vi "LABVIEW_Simulare_Adaptiv_Iluminare_Autovehicul.vi"() -> ()   [LabVIEW 2020]
panel:
  out "Volan - Faruri UNGHI":dynamicdata(graph)
  out "Viteza":dbl(graph)
  out "Grafic stari faza lunga/scurta":i32(graph)
  out "Grafic stari lumini ceata":i32(graph)
  in  "lceata":bool
  in  "?":bool
  in  "?":bool
  in  "Checkbox pt masina fata/localitate":bool
  in  "UMIDITATE":dbl(slide) scale=0.0..100.0
  in  "VITEZA":dbl(slide) scale=0.0..250.0
  out "Pozitionare Faruri":dbl(knob) scale=60.0..120.0
  in  "flunga":bool
  in  "fscurta":bool
  in  "?":bool
  in  "VOLAN":dbl(knob) scale=45.0..135.0
  out "ceata":bool
  out "adaptiv":bool
  out "fscurta":bool
  out "flunga":bool
  out "Vitezometru":dbl(knob) scale=0.0..250.0
  # "stare 0 -  Manual     oprit\nstare 1 -  Manual     f scurta\nstare 2 -  Manual     f scurta+lunga\nstare 3 -  Automat  f scurta\nstare 4 -  Automat  f scurta+lunga"
  # "stare 0 -  Oprit   \nstare 1 -  Manual\nstare 2 -  Automat"
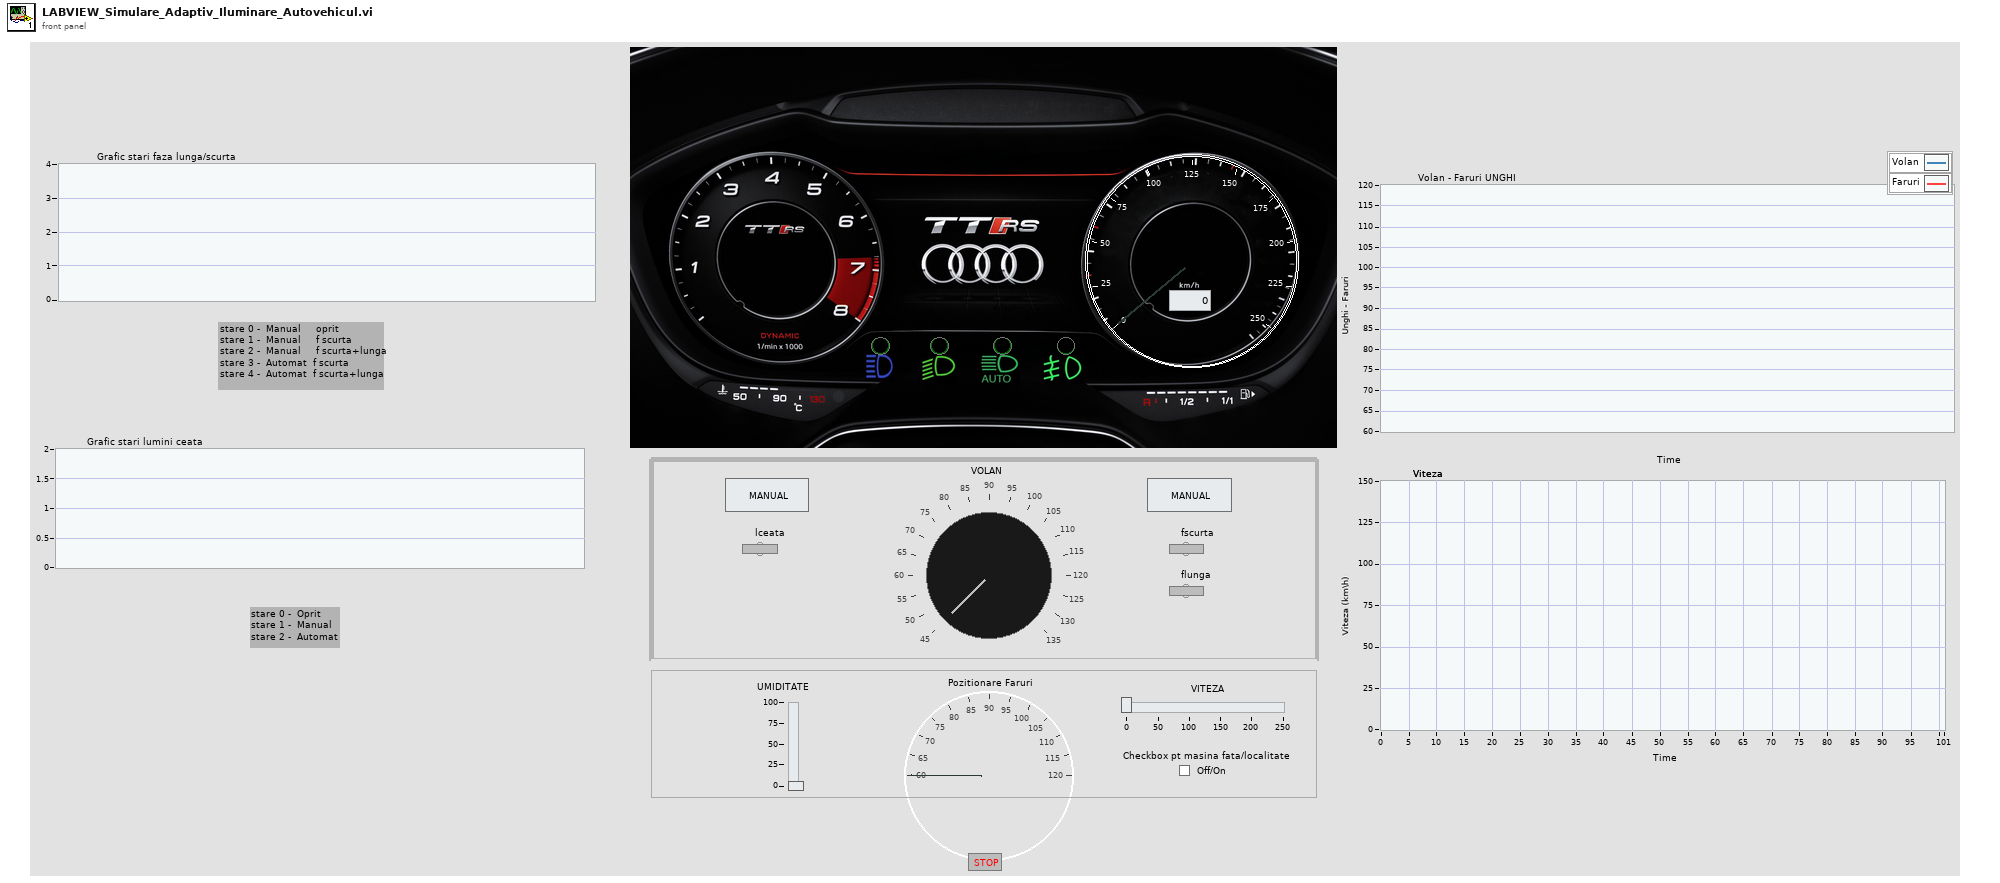
[diagram p1: front panel]
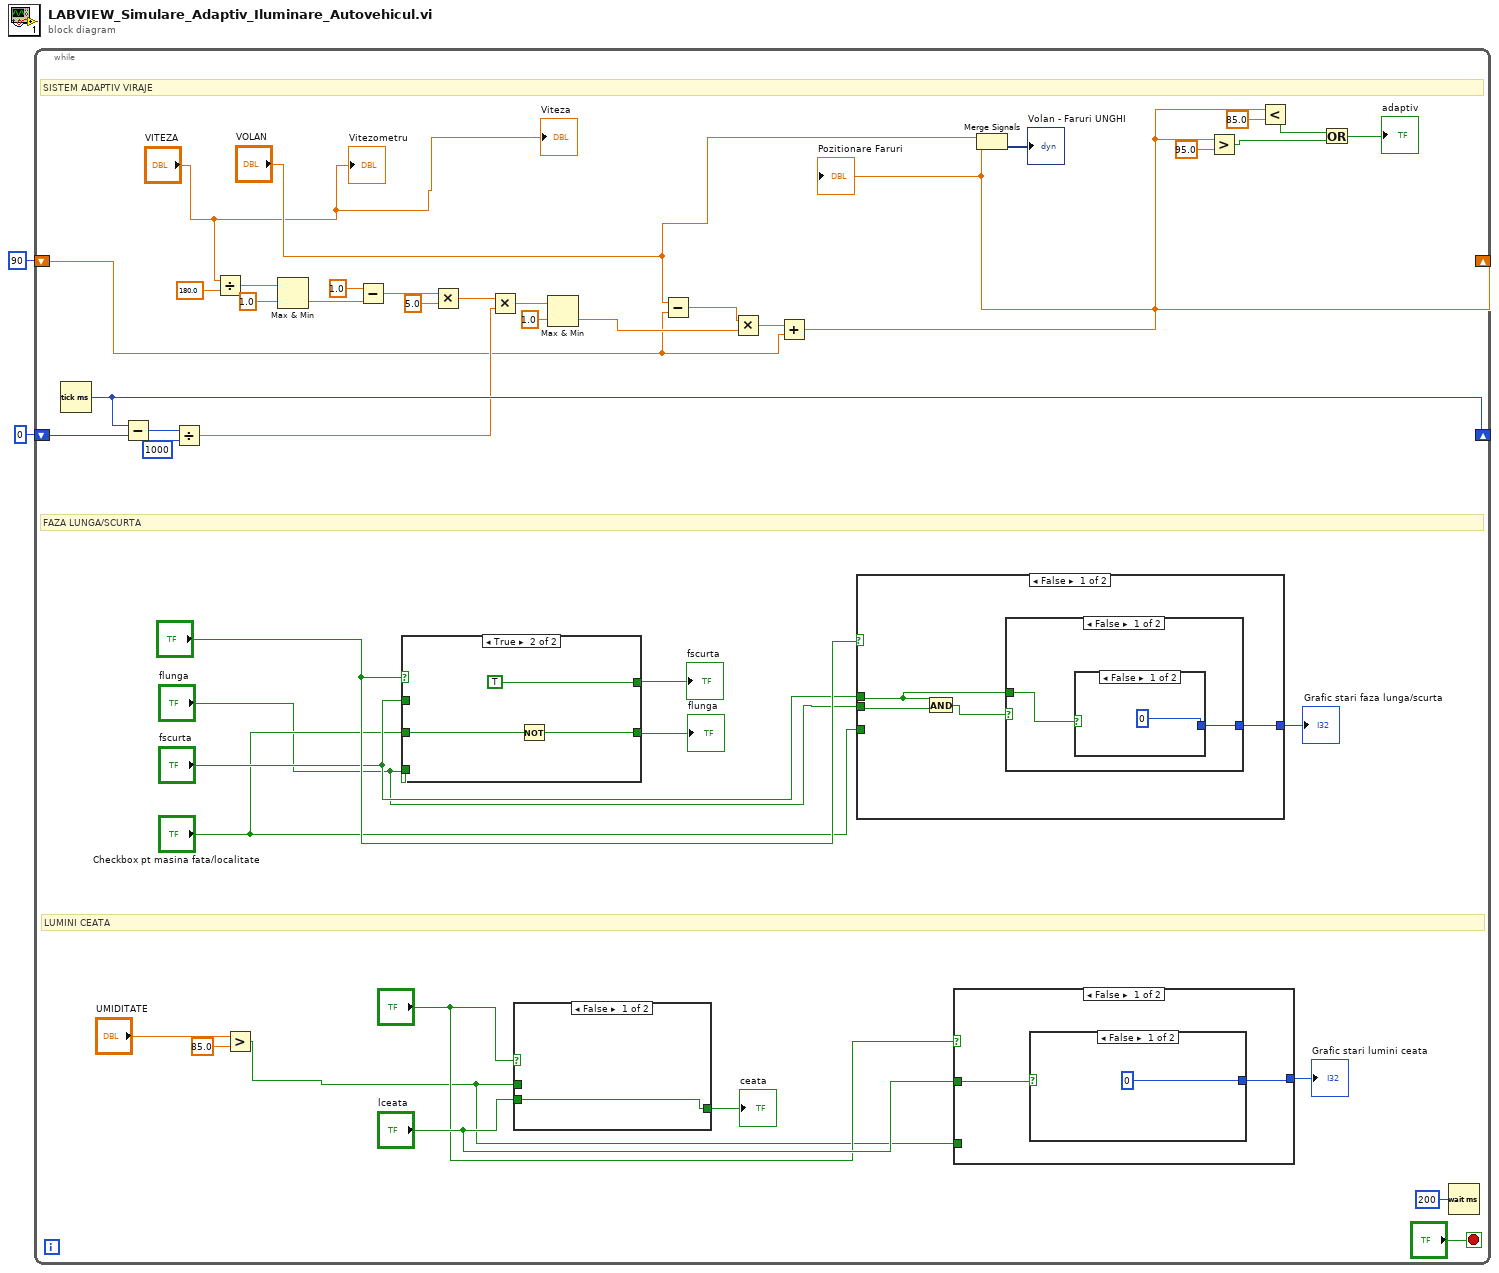
[diagram p0: block diagram]
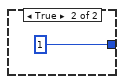
[diagram p2: hidden frame]
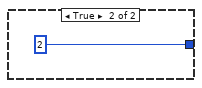
[diagram p3: hidden frame]
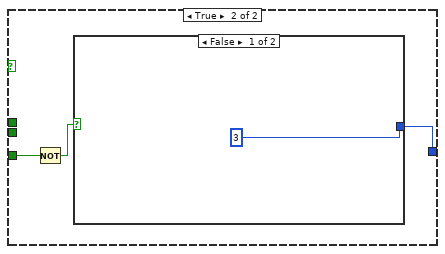
[diagram p4: hidden frame]
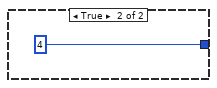
[diagram p5: hidden frame]
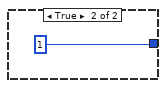
[diagram p7: hidden frame]
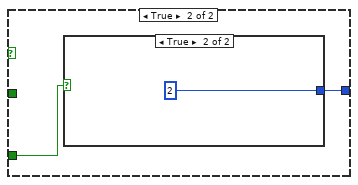
[diagram p8: hidden frame]
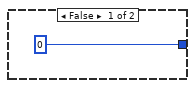
[diagram p9: hidden frame]
diagram:
  n1 = while {
    shift-right: [w6] -> _
    shift-left: 90 -> [w26]
    shift-right: [w41] -> _
    shift-left: 0 -> [w44]
    stop <- "?" stop-if-true
    # "LUMINI CEATA"
    # "FAZA LUNGA/SCURTA"
    # "SISTEM ADAPTIV VIRAJE"
    n2 = Tick Count (ms)() -> (millisecond timer value=w41:u32)
    n3 = Subtract(x=w41, y=w44) -> (x-y=w43:u32)
    n4 = Divide(x=w43, y=1000) -> (x/y=w32:dbl)
    n5 = Divide(x="VITEZA", y=180.0) -> (x/y=w39:dbl)
    n6 = Greater?(x="UMIDITATE", y=85.0) -> (0:w3:bool)
    n7 = Max & Min(x=w39, y=1.0) -> (min(x,y)=w36:dbl)  [unwired: 1 out]
    n8 = Subtract(x=1.0, y=w36) -> (x-y=w35:dbl)
    n9 = case shown="True" "?" {
      tunnel: [w62 TRUE] -> w9
      tunnel: [w61 w64] -> w8
      tunnel: "fscurta" -> [w62 _]
      tunnel: "flunga" -> [w61 _]
      tunnel: "Checkbox pt masina fata/localitate" -> [_ w63]
      frame False {
      }
      frame True {
        n10 = Not(x=w63) -> (.not. x?=w64:bool)
      }
    }
    "flunga" <- w8
    "fscurta" <- w9
    n11 = Multiply(x=w35, y=5.0) -> (x*y=w33:dbl)
    n12 = Multiply(x=w33, y=w32) -> (x*y=w31:dbl)
    n13 = case shown="False" "?" {
      tunnel: "lceata" -> [w74 _]
      tunnel: [w74 w75] -> w18
      tunnel: w3 -> [_ w75]
      frame False {
      }
      frame True {
      }
    }
    "ceata" <- w18
    n14 = Max & Min(x=w31, y=1.0) -> (min(x,y)=w28:dbl)  [unwired: 1 out]
    n15 = Subtract(x="VOLAN", y=w26) -> (x-y=w29:dbl)
    n16 = Multiply(x=w29, y=w28) -> (x*y=w27:dbl)
    n17 = Add(x=w27, y=w26) -> (x+y=w6:dbl)
    "Pozitionare Faruri" <- w6
    n18 = case shown="False" "?" {
      tunnel: "fscurta" -> [w48 _]
      tunnel: "flunga" -> [w50 _]
      tunnel: [w47 w56] -> w10
      tunnel: "Checkbox pt masina fata/localitate" -> [_ w57]
      frame False {
        n19 = And(x=w48, y=w50) -> (x .and. y?=w49:bool)
        n20 = case shown="False" w49 {
          tunnel: [w51 2] -> w47
          tunnel: w48 -> [w52 _]
          frame False {
            n21 = case shown="False" w52 {
              tunnel: [0 1] -> w51
              frame False {
              }
              frame True {
              }
            }
          }
          frame True {
          }
        }
      }
      frame True {
        n22 = Not(x=w57) -> (.not. x?=w58:bool)
        n23 = case shown="False" w58 {
          tunnel: [3 4] -> w56
          frame False {
          }
          frame True {
          }
        }
      }
    }
    "Grafic stari faza lunga/scurta" <- w10
    n24 = case shown="False" "?" {
      tunnel: [w67 w71] -> w17
      tunnel: w3 -> [_ w70]
      tunnel: "lceata" -> [w66 _]
      frame False {
        n25 = case shown="False" w66 {
          tunnel: [0 1] -> w67
          frame False {
          }
          frame True {
          }
        }
      }
      frame True {
        n26 = case shown="True" w70 {
          tunnel: [0 2] -> w71
          frame False {
          }
          frame True {
          }
        }
      }
    }
    "Grafic stari lumini ceata" <- w17
    n27 = Merge Signals("VOLAN", w6) -> (→"Volan - Faruri UNGHI":dynamicdata)
    n28 = Greater?(x=w6, y=95.0) -> (0:w22:bool)
    n29 = Less?(x=w6, y=85.0) -> (x < y?=w23:bool)
    n30 = Or(x=w23, y=w22) -> (x .or. y?=→"adaptiv":bool)
    n31 = Wait (ms)(milliseconds to wait=u32 200) -> ()  [unwired: 1 out]
    "Vitezometru" <- "VITEZA"
    "Viteza" <- "VITEZA"
  }
